vi "CropAndAverage.vi"() -> ()   [LabVIEW 2017]
uses:
  <vilib>/Utility/file.llb/Read Delimited Spreadsheet (DBL).vi
  <vilib>/Analysis/NI_AALBase.lvlib
panel:
  in  "COPY":bool
  out "Full File":string
  out "N":i32
  in  "COPY DATA":bool
  in  "Table Control":string[][](table)
  in  "STORE":bool
  out "Standard Deviation":dbl
  out "Mean":dbl
  out "Cropped Data":cluster{dbl[], dbl[]}(graph)
  out "XY Graph":cluster{"X":dbl[], "Y":dbl[]}(graph)
  in  "Path":path
  in  "STOP":bool
  in  "LOAD":bool
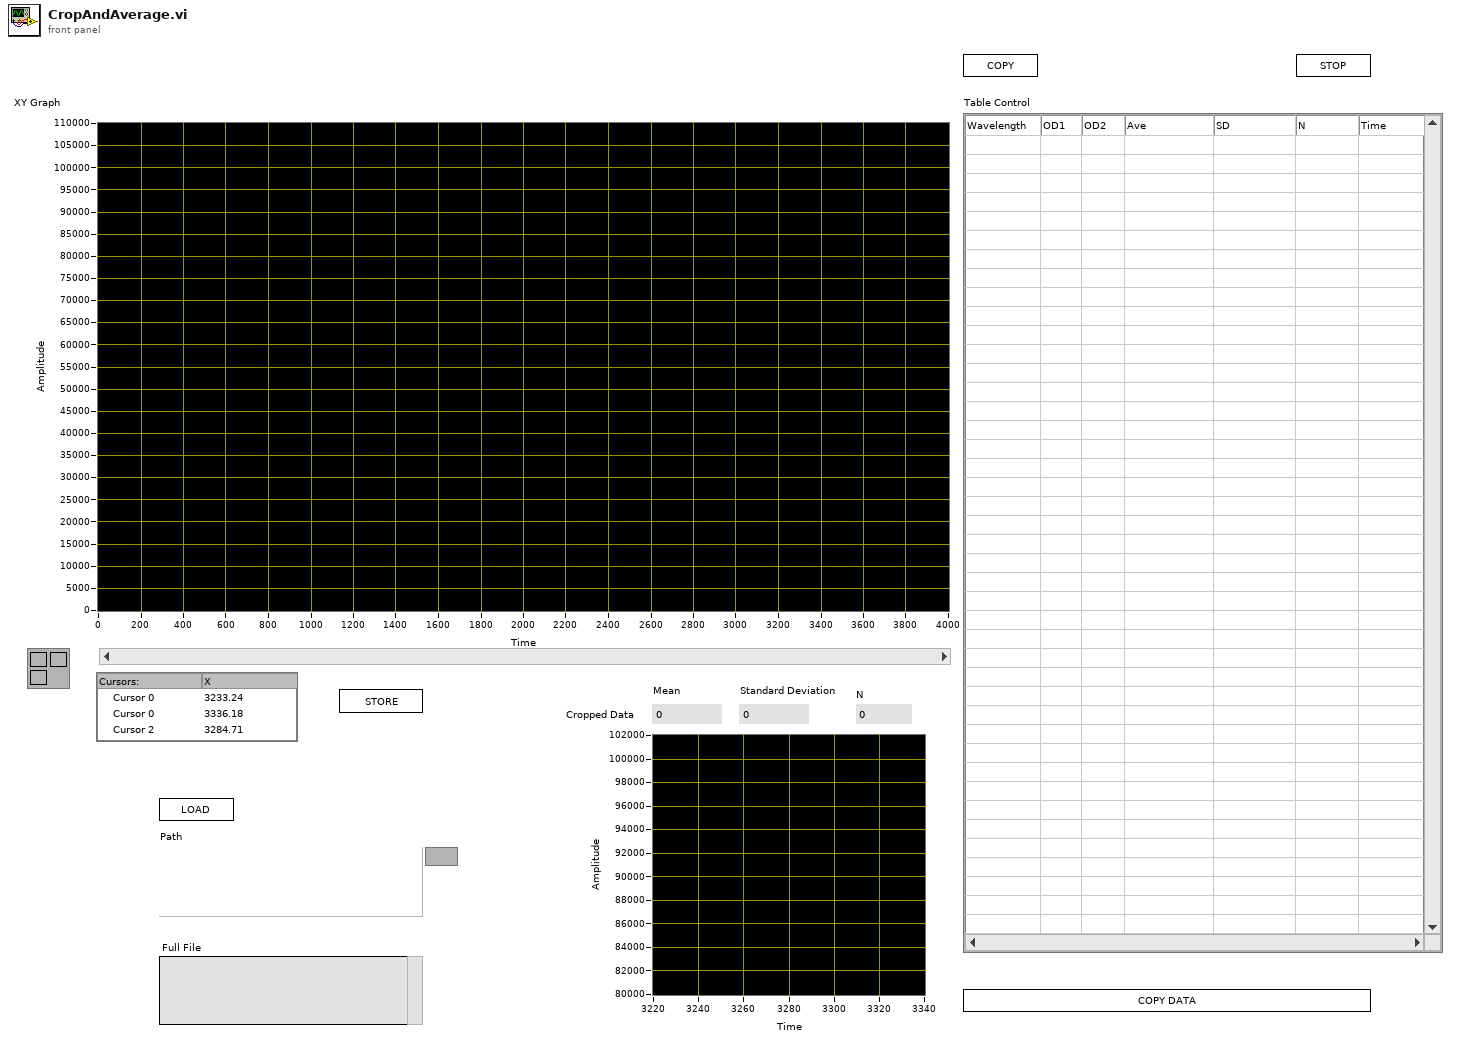
[diagram p1: front panel]
types:
  T1 = cluster{"Data":cluster{"X":dbl[], "Y":dbl[]}, "Cropped Data":cluster{"X":dbl[], "Y":dbl[]}, "Mean":dbl, "Standard Deviation":dbl, "N":dbl, "Ave Time":dbl, "index so far":i32, "Table":string[][]}
  T2 = typedef "LVCursorListTypeDef.ctl" = cluster{"Name":string, "Color":u32, "Style":u8, "Point Style":u8, "Name Visible":bool, "Allow Drag":bool, "Cursor Mode":u32, "Plot":i32, "Index":i32, "Position":cluster{"X":dbl, "Y":dbl}, "X Scale":u32, "Y Scale":u32, "Watch Plots":i32[], "Watch All Plots":bool, "Plot Area":i32, "Label Offset":cluster{"X":dbl, "Y":dbl}}[]
  T3 = cluster{"Name":string, "Color":u32, "Style":u8, "Point Style":u8, "Name Visible":bool, "Allow Drag":bool, "Cursor Mode":u32, "Plot":i32, "Index":i32, "Position":cluster{"X":dbl, "Y":dbl}, "X Scale":u32, "Y Scale":u32, "Watch Plots":i32[], "Watch All Plots":bool, "Plot Area":i32, "Label Offset":cluster{"X":dbl, "Y":dbl}}
  T4 = cluster{"Name":string, "Color":u32, "Style":u8, "Point Style":u8, "Name Visible":bool, "Allow Drag":bool, "Cursor Mode":u32, "Plot":i32, "Index":i32, "Position":cluster{"X":dbl, "Y":dbl}, "X Scale":u32, "Y Scale":u32, "Watch Plots":i32[], "Watch All Plots":bool, "Plot Area":i32, "Label Offset":cluster{"X":dbl, "Y":dbl}}[]
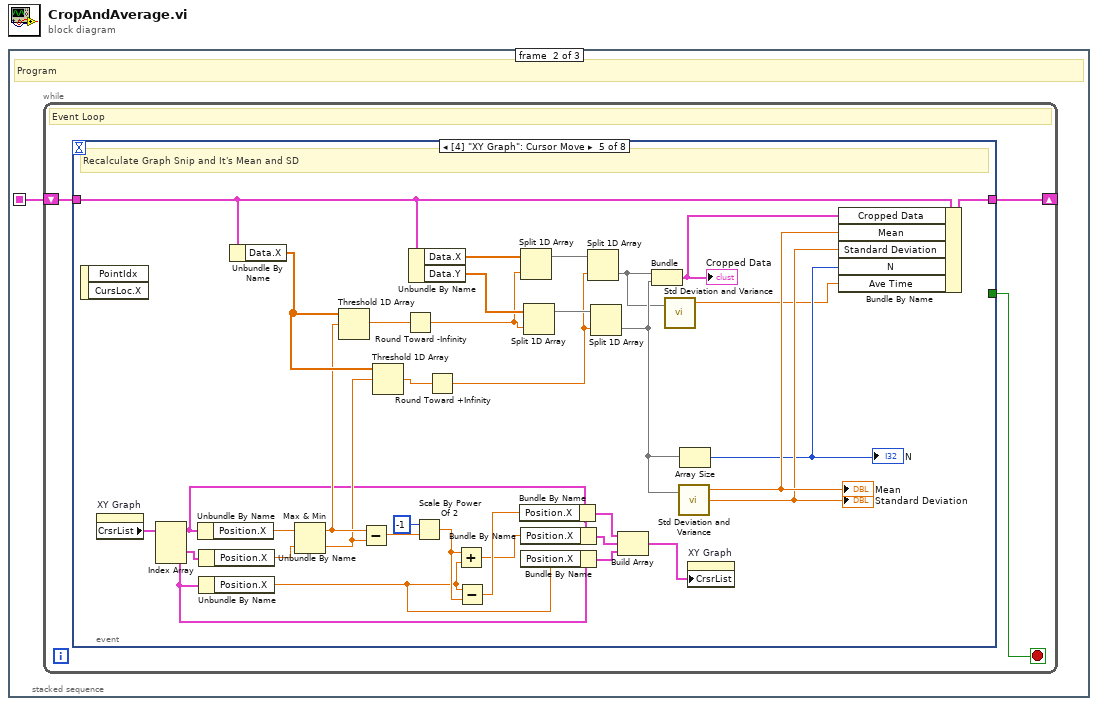
[diagram p0: block diagram]
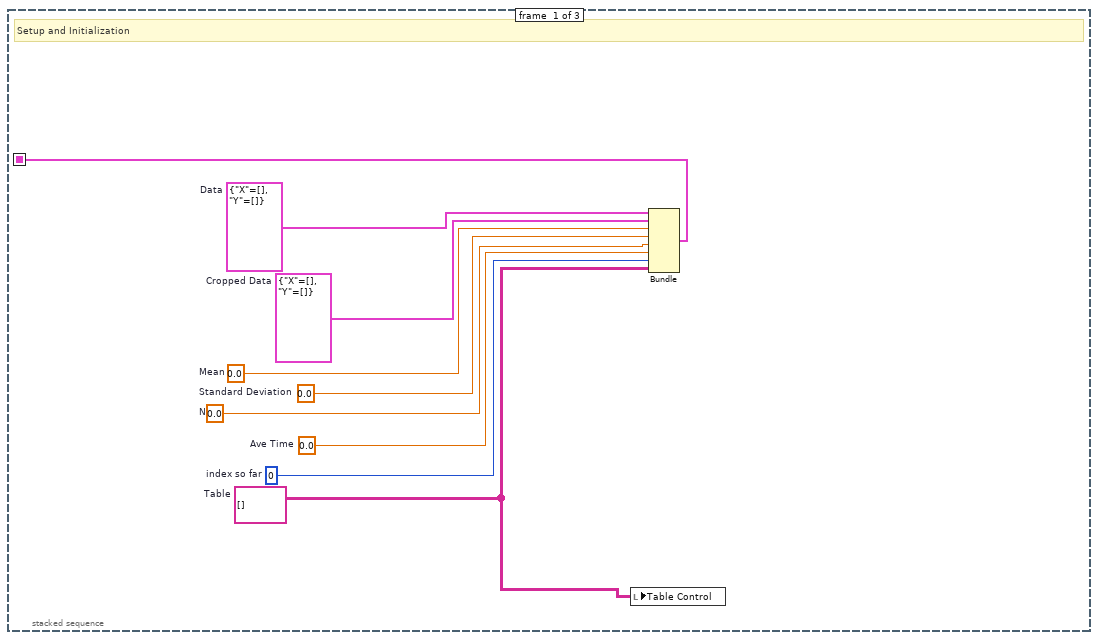
[diagram p2: hidden frame]
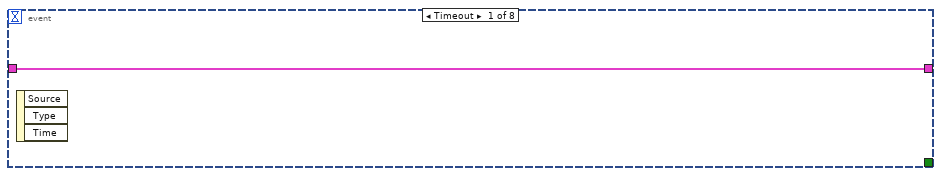
[diagram p3: hidden frame]
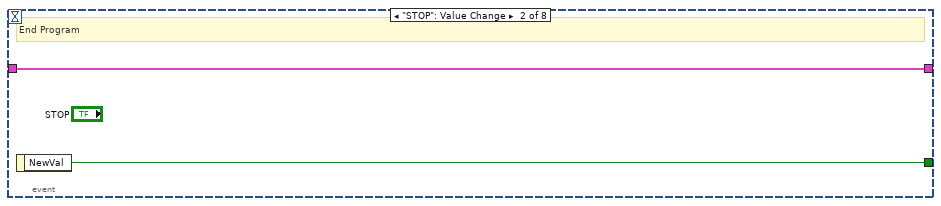
[diagram p4: hidden frame]
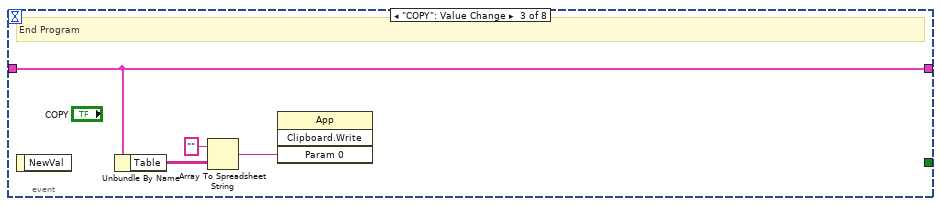
[diagram p5: hidden frame]
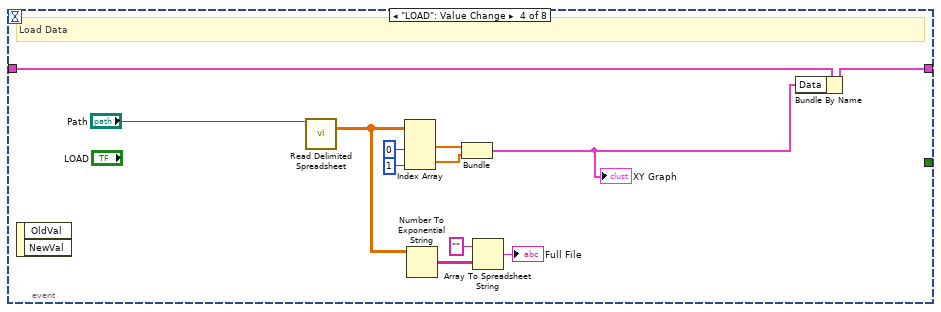
[diagram p6: hidden frame]
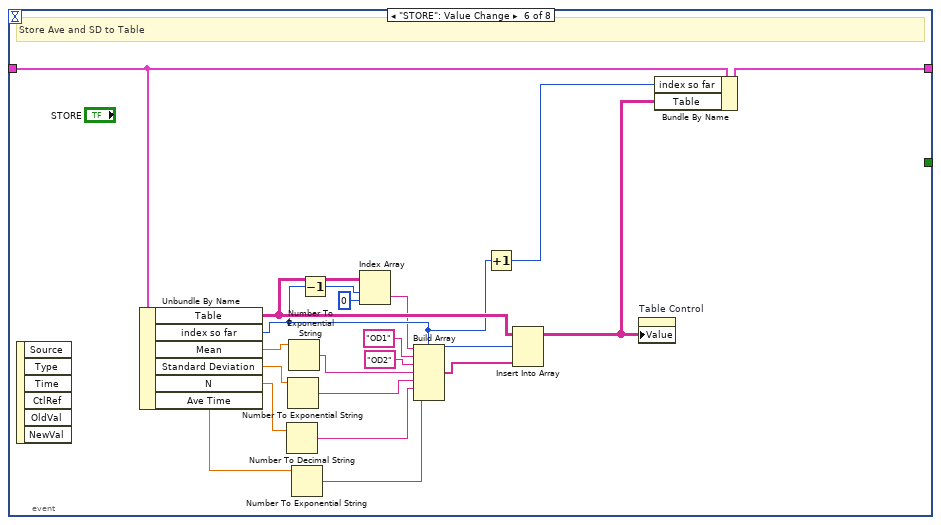
[diagram p7: hidden frame]
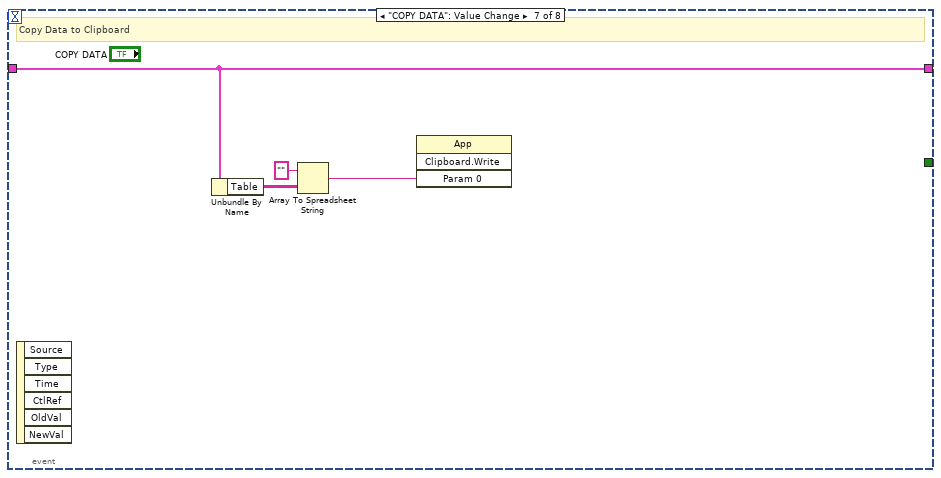
[diagram p8: hidden frame]
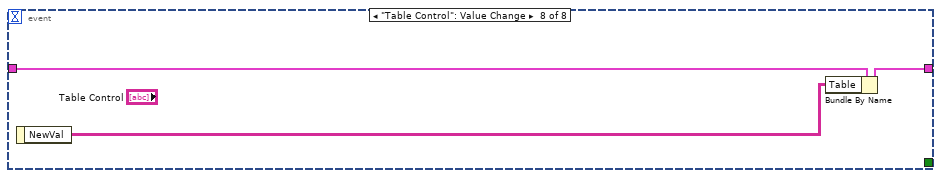
[diagram p9: hidden frame]
diagram:
  n1 = stacked-sequence {
    seq-local: [w9 _ _] -> [_ w10 _]
    frame #0 {
      w1 = 0.0  # Ave Time
      w2 = 0.0  # N
      w3 = string[][] []  # Table
      w4 = 0  # index so far
      w6 = 0.0  # Mean
      w5 = 0.0  # Standard Deviation
      w7 = cluster{"X":dbl[], "Y":dbl[]} {"X"=[], "Y"=[]}  # Cropped Data
      w8 = cluster{"X":dbl[], "Y":dbl[]} {"X"=[], "Y"=[]}  # Data
      # "Setup and Initialization"
      n2 = local write "Table Control"(w3) -> ()
      n3 = Bundle("Data"=w8, "Cropped Data"=w7, "Mean"=w6, "Standard Deviation"=w5, "N"=w2, "Ave Time"=w1, "index so far"=w4, "Table"=w3) -> (w9:T1)  [unwired: 1 in]
    }
    frame #1 {
      # "Program"
      n4 = while {
        shift-right: [w11] -> _
        shift-left: w10 -> [w12]
        stop <- w13 stop-if-true
        # "Event Loop"
        n5 = event shown="[4] \"XY Graph\": Cursor Move" {
          selector: _ -> [_ _ _ _ _ _ _ _]
          dyn-events: _ -> [_ _ _ _ _ _ _ _]
          timeout: _ -> [_ _ _ _ _ _ _ _]
          tunnel: [_ w16 _ _ _ _ _ _] -> w13
          tunnel: w12 -> [w14 w15 w18 w32 w61 w88 w92 w95]
          tunnel: [w14 w15 w18 w31 w54 w82 w92 w94] -> w11
          event Timeout {
            n6 = event-data() -> ()  [unwired: 1 in, 3 out]
          }
          event "STOP": Value Change {
            # "End Program"
            n7 = event-data() -> ("NewVal"=w16:bool)  [unwired: 1 in]
          }
          event "COPY": Value Change {
            # "End Program"
            n8 = event-data() -> ()  [unwired: 1 in, 1 out]
            n9 = Unbundle By Name(w18) -> ("Table"=w17:string[][])
            n10 = Array To Spreadsheet String(array=w17, 3:"" ("format string")) -> (spreadsheet string=w19:string)  [unwired: 1 in]
            n11 = invoke class="App" method="Clipboard.Write"("Param 0"=w19) -> ()  [unwired: 3 in, 4 out]
          }
          event "LOAD": Value Change {
            # "Load Data"
            n12 = event-data() -> ()  [unwired: 1 in, 2 out]
            n13 = call-poly <vilib>:"Read Delimited Spreadsheet.vi"("file path (dialog if empty)"="Path") -> ("all rows"=w24:dbl[][])  [unwired: 9 in, 5 out]
            n14 = Index Array(array=w24, index (col) #1=0 ("disabled index (col)"), index (col) #2=1 ("index (col)")) -> (element #1=w27:dbl[], element #2=w26:dbl[])  [unwired: 2 in]
            n15 = Number To Exponential String(number=w24) -> (E-format string=w23:string[][])  [unwired: 3 in]
            n16 = Bundle("all rows"=w27, "all rows"=w26) -> (w25:cluster{"all rows":dbl[], "all rows":dbl[]})  [unwired: 1 in]
            "XY Graph" <- w25
            n17 = Array To Spreadsheet String(array=w23, 3:"" ("format string")) -> (spreadsheet string=→"Full File":string)  [unwired: 1 in]
            n18 = Bundle By Name(cluster=w32, "Data"=w25) -> (w31:T1)
          }
          event "XY Graph": Cursor Move {
            # "Recalculate Graph Snip and It's Mean and SD"
            n19 = event-data() -> ()  [unwired: 1 in, 2 out]
            n20 = property on="XY Graph" class="XYGraph (strict)"() -> ("CrsrList"=w68:T2)  [unwired: 2 in, 2 out]
            n21 = Index Array(array=w68) -> (element #1=w40:T3, element #2=w67:T3, element #3=w41:T3)  [unwired: 3 in]
            n22 = Unbundle By Name(w40) -> ("Position.X"=w66:dbl)
            n23 = Unbundle By Name(w67) -> ("Position.X"=w65:dbl)
            n24 = Unbundle By Name(w41) -> ("Position.X"=w37:dbl)
            n25 = Unbundle By Name(w61) -> ("Data.X"=w64:dbl[])
            n26 = Max & Min(x=w66, y=w65) -> (max(x,y)=w46:dbl, min(x,y)=w45:dbl)
            n27 = Threshold 1D Array(2:w46, 3:w64) -> (0:w62:dbl)  [unwired: 1 in]
            n28 = Subtract(x=w46, y=w45) -> (x-y=w44:dbl)
            n29 = Threshold 1D Array(2:w45, 3:w64) -> (0:w63:dbl)  [unwired: 1 in]
            n30 = Round Toward -Infinity(1:w62) -> (0:w56:dbl)
            n31 = Unbundle By Name(w61) -> ("Data.X"=w60:dbl[], "Data.Y"=w58:dbl[])
            n32 = Scale By Power Of 2(n=i16 -1, x=w44) -> (x*2^n=w42:dbl)
            n33 = Round Toward +Infinity(x=w63) -> (ceil(x): smallest int >= x=w55:dbl)
            n34 = Add(x=w42, y=w37) -> (x+y=w38:dbl)
            n35 = Subtract(x=w37, y=w42) -> (x-y=w39:dbl)
            n36 = Bundle By Name(cluster=w40, "Position.X"=w39) -> (w36:T3)
            n37 = Split 1D Array(array=w60, index=w56) -> (first subarray=w59:dbl[])  [unwired: 1 out]
            n38 = Bundle By Name(cluster=w40, "Position.X"=w38) -> (w35:T3)
            n39 = Bundle By Name(cluster=w41, "Position.X"=w37) -> (w34:T3)
            n40 = Split 1D Array(array=w58, index=w56) -> (first subarray=w57:dbl[])  [unwired: 1 out]
            n41 = Split 1D Array(array=w59, index=w55) -> (second subarray=w48:dbl[])  [unwired: 1 out]
            n42 = Split 1D Array(array=w57, index=w55) -> (second subarray=w50:dbl[])  [unwired: 1 out]
            n43 = Build Array(w36, w35, w34) -> (w33:T4)
            n44 = Bundle(w48, w50) -> (w53:cluster{dbl[], dbl[]})  [unwired: 1 in]
            "Cropped Data" <- w53
            n45 = call <vilib>:"Std Deviation and Variance.vi"("X"=w48) -> ("mean"=w47:dbl)  [unwired: 1 in, 2 out]
            n46 = call <vilib>:"Std Deviation and Variance.vi"("X"=w50) -> ("mean"=w52:dbl, "standard deviation"=w51:dbl)  [unwired: 1 in, 1 out]
            "Mean" <- w52
            "Standard Deviation" <- w51
            n47 = Array Size(array=w50) -> (size(s)=w49:i32)
            "N" <- w49
            n48 = property on="XY Graph" class="XYGraph (strict)"("CrsrList"=w33) -> ()  [unwired: 2 in, 2 out]
            n49 = Bundle By Name(cluster=w61, "Cropped Data"=w53, "Mean"=w52, "Standard Deviation"=w51, "N"=w49, "Ave Time"=w47) -> (w54:T1)
          }
          event "STORE": Value Change {
            # "Store Ave and SD to Table"
            n50 = event-data() -> ()  [unwired: 1 in, 6 out]
            n51 = Unbundle By Name(w88) -> ("Table"=w77:string[][], "index so far"=w75:i32, "Mean"=w86:dbl, "Standard Deviation"=w87:dbl, "N"=w72:dbl, "Ave Time"=w70:dbl)
            n52 = Number To Decimal String(number=w72) -> (decimal integer string=w71:string)  [unwired: 1 in]
            n53 = Number To Exponential String(number=w87) -> (E-format string=w84:string)  [unwired: 3 in]
            n54 = Number To Exponential String(number=w86) -> (E-format string=w85:string)  [unwired: 3 in]
            n55 = Number To Exponential String(number=w70) -> (E-format string=w69:string)  [unwired: 3 in]
            n56 = Decrement(x=w75) -> (x-1=w74:i32)
            n57 = Index Array(array=w77, index (row)=w74, index (col)=0 ("disabled index (col)")) -> (element=w73:string)
            n58 = Build Array(w73, "OD1" ("format string"), "OD2" ("format string"), w85, w84, w71, w69) -> (w83:string[])
            n59 = Increment(x=w75) -> (x+1=w80:i32)
            n60 = Insert Into Array(array=w77, index (row)=w75, new element=w83) -> (w81:string[][])  [unwired: 1 in]
            n61 = property on="Table Control" class="Tbl (strict)"("Value"=w81) -> ()  [unwired: 2 in, 2 out]
            n62 = Bundle By Name(cluster=w88, "index so far"=w80, "Table"=w81) -> (w82:T1)
          }
          event "COPY DATA": Value Change {
            # "Copy Data to Clipboard"
            n63 = event-data() -> ()  [unwired: 1 in, 6 out]
            n64 = Unbundle By Name(w92) -> ("Table"=w91:string[][])
            n65 = Array To Spreadsheet String(array=w91, 3:"" ("format string")) -> (spreadsheet string=w90:string)  [unwired: 1 in]
            n66 = invoke class="App" method="Clipboard.Write"("Param 0"=w90) -> ()  [unwired: 3 in, 4 out]
          }
          event "Table Control": Value Change {
            n67 = event-data() -> ("NewVal"=w93:string[][])  [unwired: 1 in]
            n68 = Bundle By Name(cluster=w95, "Table"=w93) -> (w94:T1)
          }
        }
      }
    }
    frame #2 {
      # "Cleanup and Shutdown"
    }
  }
